vi "svfa_Scaled Time Domain Window (dual).vi"(0 "Signal in [X]":waveform(dbl)={"t0"=timestamp(0 s since 1904-01-01), "dt"=1.953125e-05, "Y"=[]}, 1 "processing control":T2(ring), 5 "Signal in [Y]":waveform(dbl)={"t0"=timestamp(0 s since 1904-01-01), "dt"=1.953125e-05, "Y"=[]}, 7 "window":T1 items=["None"=0, "Hanning"=1, "Hamming"=2, "Blackman-Harris"=3, "Exact Blackman"=4, "Blackman"=5, "Flat Top"=6, "4 Term B-Harris "=7, "7 Term B-Harris"=8, "Low Sidelobe"=9, "Force - Exponential"=10, "Blackman Nuttall"=11, "Triangle"=30, "Bartlett-Hanning"=31, "Bohman"=32, "Parzen"=33, "Welch"=34, "Kaiser"=60, "Dolph-Chebyshev"=61, "Gaussian"=62], 9 "force/exp settings":T3={"force window [%]"=50.0, "exp window [%]"=10.0} {"exp window [%]" min=0.0 max=100.0 format="%.2f"; "force window [%]" min=0.0 max=100.0 format="%.2f"}, 11 "error in (no error)":errorcluster) -> (3 "dup processing control":T2(ring), 4 "Windowed signal [X]":waveform(dbl)={"t0"=timestamp(0 s since 1904-01-01), "dt"=1.953125e-05, "Y"=[]}, 6 "Windowed signal [Y]":waveform(dbl)={"t0"=timestamp(0 s since 1904-01-01), "dt"=1.953125e-05, "Y"=[]}, 8 "window":T1 items=["None"=0, "Hanning"=1, "Hamming"=2, "Blackman-Harris"=3, "Exact Blackman"=4, "Blackman"=5, "Flat Top"=6, "4 Term B-Harris "=7, "7 Term B-Harris"=8, "Low Sidelobe"=9, "Force - Exponential"=10, "Blackman Nuttall"=11, "Triangle"=30, "Bartlett-Hanning"=31, "Bohman"=32, "Parzen"=33, "Welch"=34, "Kaiser"=60, "Dolph-Chebyshev"=61, "Gaussian"=62], 10 "window size":i32, 13 "window constants":cluster{"eq noise BW":dbl, "coherent gain":dbl} {"coherent gain" format="%.2f"; "eq noise BW" format="%.2f"}, 15 "error out":errorcluster)   [LabVIEW 2017]
doc: "Applies the selected window to the time-domain signal. The VI scales the result so that when the power or amplitude spectrum of the windowed waveform is computed, all windows provide the same level within the accuracy constraints of the window."
uses:
  <vilib>/addons/_NISVFA/_Shared subVIs/Controls/svc_Window [Dual FFT].ctl
  <vilib>/addons/_NISVFA/_Shared subVIs/Windowing/svfa_Scaled Time Domain Window (Array).vi
  <vilib>/Analysis/4window.llb/Force Window.vi
  <vilib>/Analysis/4window.llb/Force Window (DBL).vi
  <vilib>/Analysis/4window.llb/Exponential Window.vi
  <vilib>/Analysis/4window.llb/Exponential Window (DBL).vi
  <vilib>/Utility/error.llb/Error Cluster From Error Code.vi
  <vilib>/Analysis/0measdsp.llb/Scaled Time Domain Window.vi
  <vilib>/Analysis/0measdsp.llb/Scaled Time Domain Window (DBL).vi
  <vilib>/addons/_NISVFA/_Spectrum Processing/subVIs/svfa_Spectrum Info Window to windowTd Type Def.vi
  <vilib>/addons/_NISVFA/_Shared subVIs/Common/svc_Window Parameters.vi
  <vilib>/addons/_NISVFA/_Shared subVIs/Common/svc_Get Window Info.vi
panel:
  # "Scaled Time Domain Window"
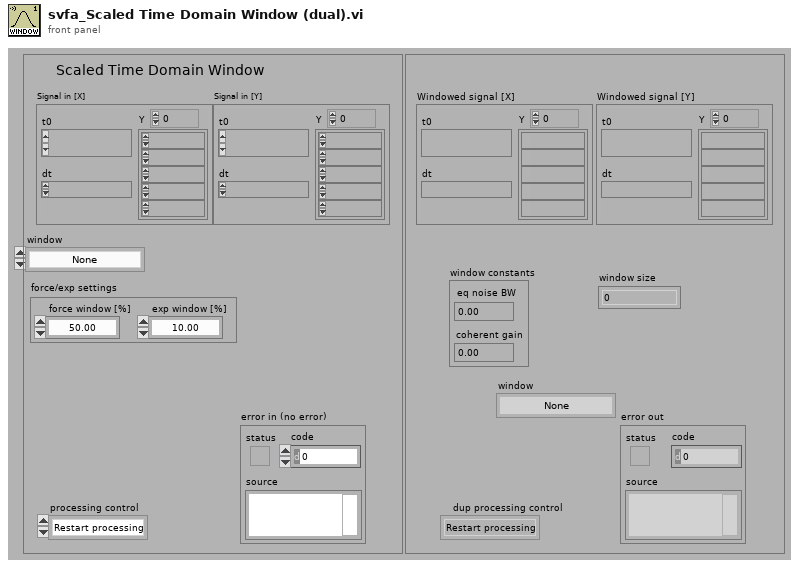
[diagram p1: front panel]
types:
  T1 = typedef "svc_Window [Dual FFT].ctl" = u32
  T2 = enum16{"Restart processing", "Continue processing", "Skip processing"}
  T3 = cluster{"force window [%]":dbl, "exp window [%]":dbl}
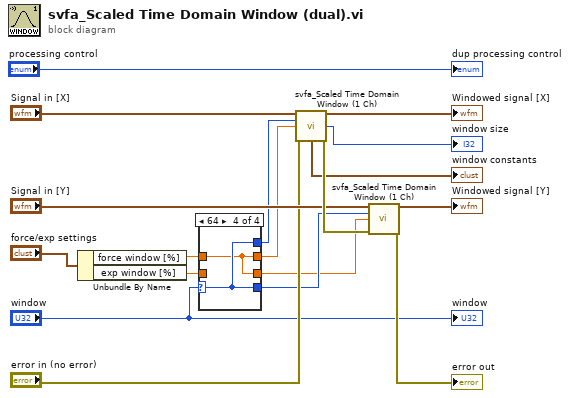
[diagram p0: block diagram]
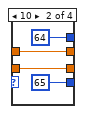
[diagram p3: hidden frame]
diagram:
  n1 = Unbundle By Name("force/exp settings") -> ("force window [%]"=w8:dbl, "exp window [%]"=w7:dbl)
  n2 = case shown="64" "window" {
    selector: "window" -> [w21 _ w27 w29]
    tunnel: [w21 u16 64 ("window") w27 w29] -> w5
    tunnel: [w21 u16 65 ("window") w27 w29] -> w4
    tunnel: [w20 w23 w26 w28] -> w3
    tunnel: w8 -> [w20 w23 _ w28]
    tunnel: [w19 w22 w26 w28] -> w2
    tunnel: w7 -> [w19 w22 w26 _]
    frame 0, Default {
    }
    frame 10 {
    }
    frame 65 {
    }
    frame 64 {
    }
  }
  n3 = call <vilib>:"svfa_Scaled Time Domain Window (1 Ch).vi"("Signal in [X]"="Signal in [X]", "window"=w5, "window parameter"=w3, "error in"="error in (no error)") -> ("Windowed Waveform"=→"Windowed signal [X]":waveform(dbl), "window length"=→"window size":i32, "window constants"=→"window constants":cluster{"ENBW":dbl, "CG":dbl}, "error out"=w17:errorcluster)  [unwired: 6 in, 2 out]
  n4 = call <vilib>:"svfa_Scaled Time Domain Window (1 Ch).vi"("Signal in [X]"="Signal in [Y]", "window"=w4, "window parameter"=w2, "error in"=w17) -> ("Windowed Waveform"=→"Windowed signal [Y]":waveform(dbl), "error out"=→"error out":errorcluster)  [unwired: 6 in, 4 out]
  "dup processing control" <- "processing control"
  "window" <- "window"
